vi "Lidar_거리 필터.vi"() -> ()   [LabVIEW 2016]
panel:
  in  "필터 거리(쉬프트 값보다 크게)":dbl=2500.0
  in  "행 개수":i32=721
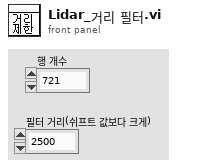
[diagram p1: front panel]
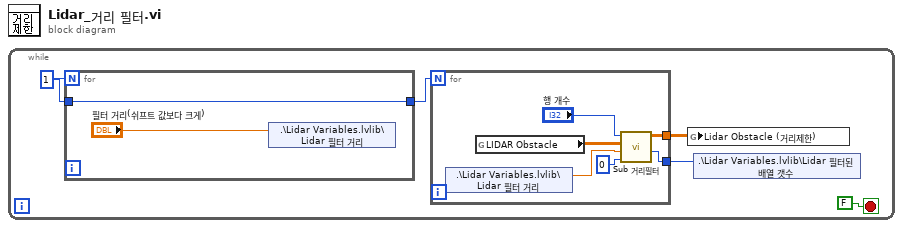
[diagram p0: block diagram]
diagram:
  n1 = while {
    stop <- FALSE stop-if-true
    w4 = 1
    n2 = for {
      N: w4 -> [_]
      tunnel: w4 -> [w13]
      tunnel: [w13] -> w5
      n3 = shared-variable ".\\Lidar Variables.lvlib\\Lidar 필터 거리"("필터 거리(쉬프트 값보다 크게)") -> ()  [unwired: 1 in, 1 out]
    }
    n4 = for {
      N: w5 -> [_]
      tunnel: [w7] -> w2
      tunnel: [w6] -> w1
      n5 = shared-variable ".\\Lidar Variables.lvlib\\Lidar 필터 거리"() -> (w11:dbl)  [unwired: 1 in, 1 out]
      n6 = global read "[GV]_Lidar Obstacle.vi" "LIDAR Obstacle"() -> (w9:dbl[][])
      n7 = call "Sub 거리필터.vi"("거리 데이터 열"=0, "필터 거리(쉬프트 값보다 크게)"=w11, "입력 배열(2차원)"=w9, "행 수"="행 개수") -> ("거리필터된 갯수"=w6:i32, "거리 필터된 배열"=w7:dbl[][])  [unwired: 6 in]
    }
    n8 = global write "[GV]_Lidar Obstacle (거리제한).vi" "Lidar Obstacle (거리제한)"(w2) -> ()
    n9 = shared-variable ".\\Lidar Variables.lvlib\\Lidar 필터된 배열 갯수"(w1) -> ()  [unwired: 1 in, 1 out]
  }
